vi "rtLoad.vi"(8 "WOB Zero In":dbl format="%#_13g", 9 "Zero":bool, 10 "Load 2: Voltage (v)":dbl, 11 "Load 1: Voltage (V)":dbl) -> (0 "WOB Zero Out":dbl, 1 "Total Force (lbf)":dbl, 2 "Load 2: Force (lbf)":dbl, 3 "Load 1: Force (lbf)":dbl)   [LabVIEW 2019]
panel:
  # "READ WOB Sensors"
  # "Futek LCM375 10klbf Tension"
  # "S/N 702360 Calibration Data"
  # "S/N 702359 Calibration Data"
  # "L1 Excitation = 9.99 Vdc"
  # "L2 Excitation = 9.99 Vdc"
  # "L1 Calib Pt -1 (<0) = 2.1364e-4 lbf/(mV/V)"
  # "L2 Calib Pt -1 (<0) = 2.1316e-4 lbf/(mV/V)"
  # "L1 Calib Pt 0 (0-2k) = 2.1515e-4 lbf/(mV/V)"
  # "L2 Calib Pt 0 (0-2k) = 2.1370e-4 lbf/(mV/V)"
  # "L1 Calib Pt 1 (2k-4k) = 2.1560e-4 lbf/(mV/V)"
  # "L2 Calib Pt 1 (2k-4k) = 2.1445e-4 lbf/(mV/V)"
  # "L1 Calib Pt 2 (4k-6k) = 2.1585e-4 lbf/(mV/V)"
  # "L2 Calib Pt 2 (4k-6k) = 2.1505e-4 lbf/(mV/V)"
  # "L1 Calib Pt 3 (6k-8k) = 2.1685e-4 lbf/(mV/V)"
  # "L2 Calib Pt 3 (6k-8k) = 2.1525e-4 lbf/(mV/V)"
  # "L1 Calib Pt 4 (8k-10k) = 2.1566e-4 lbf/(mV/V)"
  # "L2 Calib Pt 4 (8k-10k) = 2.1620e-4 lbf/(mV/V)"
  # "L1 Factory Zero = 0.0044 mV/V"
  # "L2 Factory Zero = 0.0043 mV/V"
  # "L1 Nominal Zero = 0.00667 mV/V"
  # "L2 Nominal Zero = 0.00572 mV/V"
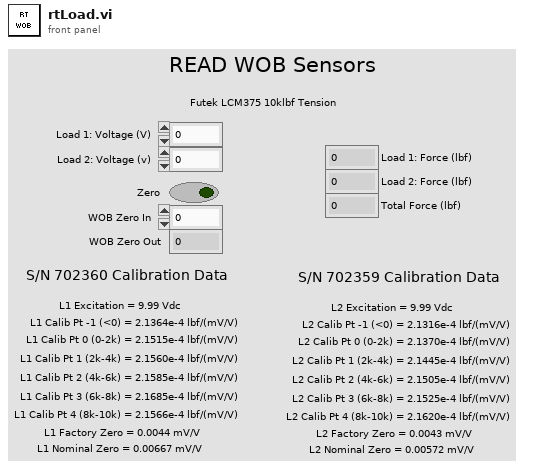
[diagram p1: front panel]
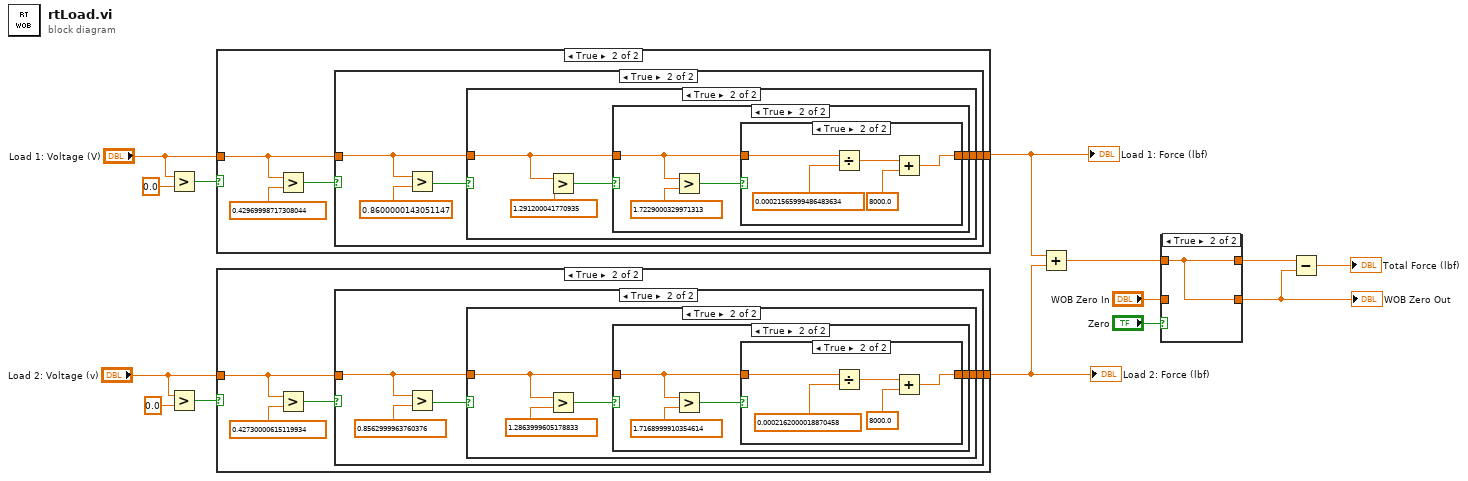
[diagram p0: block diagram]
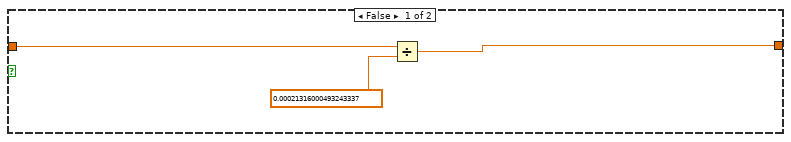
[diagram p3: hidden frame]
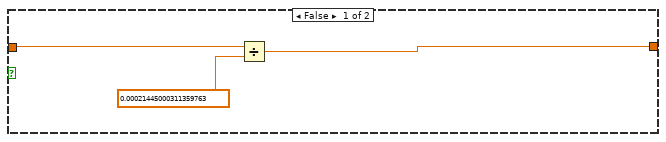
[diagram p4: hidden frame]
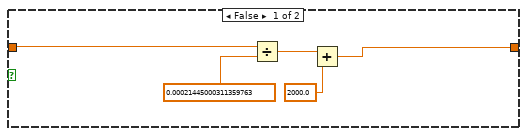
[diagram p5: hidden frame]
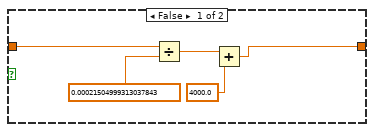
[diagram p6: hidden frame]
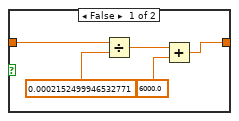
[diagram p7: hidden frame]
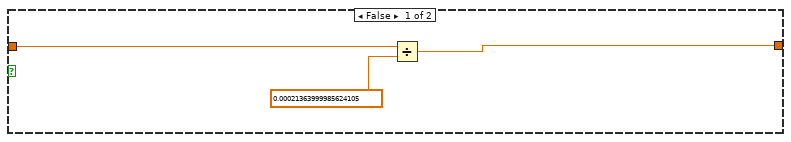
[diagram p8: hidden frame]
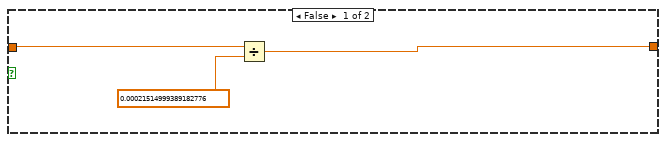
[diagram p9: hidden frame]
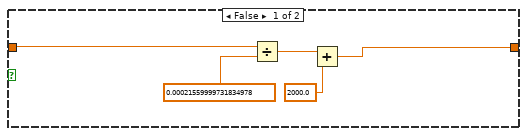
[diagram p10: hidden frame]
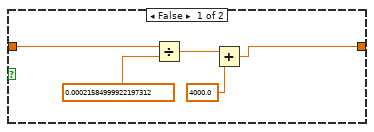
[diagram p11: hidden frame]
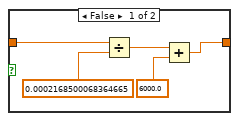
[diagram p12: hidden frame]
diagram:
  n1 = Greater?(x="Load 1: Voltage (V)", y=0.0) -> (0:w11:bool)
  n2 = Greater?(x="Load 2: Voltage (v)", y=0.0) -> (0:w14:bool)
  n3 = case shown="True" w11 {
    tunnel: "Load 1: Voltage (V)" -> [w16 w21]
    tunnel: [w15 w18] -> w7
    frame False {
      n4 = Divide(x=w16, y=sgl 0.00021364) -> (x/y=w15:dbl)
    }
    frame True {
      n5 = Greater?(x=w21, y=sgl 0.4297) -> (0:w20:bool)
      n6 = case shown="True" w20 {
        tunnel: w21 -> [w23 w26]
        tunnel: [w22 w25] -> w18
        frame False {
          n7 = Divide(x=w23, y=sgl 0.00021515) -> (x/y=w22:dbl)
        }
        frame True {
          n8 = Greater?(x=w26, y=sgl 0.86) -> (0:w27:bool)
          n9 = case shown="True" w27 {
            tunnel: w26 -> [w29 w34]
            tunnel: [w31 w35] -> w25
            frame False {
              n10 = Divide(x=w29, y=sgl 0.0002156) -> (x/y=w33:dbl)
              n11 = Add(x=w33, y=sgl 2000.0) -> (x+y=w31:dbl)
            }
            frame True {
              n12 = Greater?(x=w34, y=sgl 1.2912) -> (0:w36:bool)
              n13 = case shown="True" w36 {
                tunnel: w34 -> [w39 w43]
                tunnel: [w38 w44] -> w35
                frame False {
                  n14 = Divide(x=w39, y=sgl 0.00021585) -> (x/y=w42:dbl)
                  n15 = Add(x=w42, y=sgl 4000.0) -> (x+y=w38:dbl)
                }
                frame True {
                  n16 = Greater?(x=w43, y=sgl 1.7229) -> (0:w45:bool)
                  n17 = case shown="True" w45 {
                    tunnel: w43 -> [w48 w56]
                    tunnel: [w47 w52] -> w44
                    frame False {
                      n18 = Divide(x=w48, y=sgl 0.00021685) -> (x/y=w51:dbl)
                      n19 = Add(x=w51, y=sgl 6000.0) -> (x+y=w47:dbl)
                    }
                    frame True {
                      n20 = Divide(x=w56, y=sgl 0.00021566) -> (x/y=w54:dbl)
                      n21 = Add(x=w54, y=sgl 8000.0) -> (x+y=w52:dbl)
                    }
                  }
                }
              }
            }
          }
        }
      }
    }
  }
  "Load 1: Force (lbf)" <- w7
  n22 = case shown="True" w14 {
    tunnel: "Load 2: Voltage (v)" -> [w58 w63]
    tunnel: [w57 w60] -> w6
    frame False {
      n23 = Divide(x=w58, y=sgl 0.00021316) -> (x/y=w57:dbl)
    }
    frame True {
      n24 = Greater?(x=w63, y=sgl 0.4273) -> (0:w62:bool)
      n25 = case shown="True" w62 {
        tunnel: w63 -> [w65 w68]
        tunnel: [w64 w67] -> w60
        frame False {
          n26 = Divide(x=w65, y=sgl 0.00021445) -> (x/y=w64:dbl)
        }
        frame True {
          n27 = Greater?(x=w68, y=sgl 0.8563) -> (0:w69:bool)
          n28 = case shown="True" w69 {
            tunnel: w68 -> [w71 w76]
            tunnel: [w73 w77] -> w67
            frame False {
              n29 = Divide(x=w71, y=sgl 0.00021445) -> (x/y=w75:dbl)
              n30 = Add(x=w75, y=sgl 2000.0) -> (x+y=w73:dbl)
            }
            frame True {
              n31 = Greater?(x=w76, y=sgl 1.2864) -> (0:w78:bool)
              n32 = case shown="True" w78 {
                tunnel: w76 -> [w81 w85]
                tunnel: [w80 w86] -> w77
                frame False {
                  n33 = Divide(x=w81, y=sgl 0.00021505) -> (x/y=w84:dbl)
                  n34 = Add(x=w84, y=sgl 4000.0) -> (x+y=w80:dbl)
                }
                frame True {
                  n35 = Greater?(x=w85, y=sgl 1.7169) -> (0:w87:bool)
                  n36 = case shown="True" w87 {
                    tunnel: w85 -> [w90 w98]
                    tunnel: [w89 w94] -> w86
                    frame False {
                      n37 = Divide(x=w90, y=sgl 0.00021525) -> (x/y=w93:dbl)
                      n38 = Add(x=w93, y=sgl 6000.0) -> (x+y=w89:dbl)
                    }
                    frame True {
                      n39 = Divide(x=w98, y=sgl 0.0002162) -> (x/y=w96:dbl)
                      n40 = Add(x=w96, y=sgl 8000.0) -> (x+y=w94:dbl)
                    }
                  }
                }
              }
            }
          }
        }
      }
    }
  }
  "Load 2: Force (lbf)" <- w6
  n41 = Add(x=w7, y=w6) -> (x+y=w3:dbl)
  n42 = case shown="True" "Zero" {
    tunnel: "WOB Zero In" -> [w100 _]
    tunnel: w3 -> [w99 w101]
    tunnel: [w100 w101] -> w2
    tunnel: [w99 w101] -> w1
    frame False {
    }
    frame True {
    }
  }
  "WOB Zero Out" <- w2
  n43 = Subtract(x=w1, y=w2) -> (x-y=→"Total Force (lbf)":dbl)
